vi "Ex3_BlinkingSignalLights.vi"() -> ()   [LabVIEW 2024]
panel:
  out "Array":bool[](array[boolean])
  in  "Boolean":bool
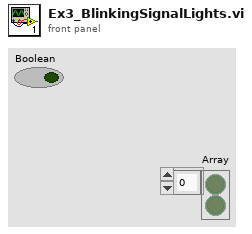
[diagram p1: front panel]
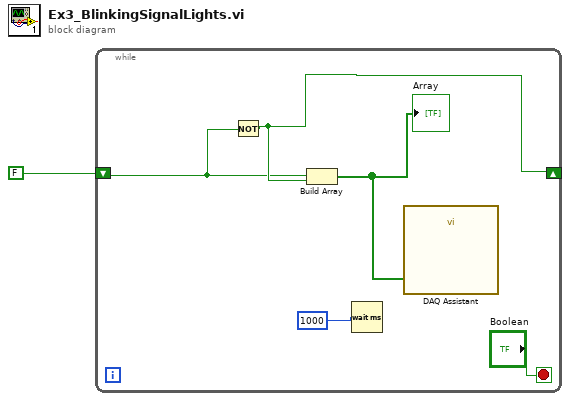
[diagram p0: block diagram]
diagram:
  n1 = while {
    shift-right: [w4] -> _
    shift-left: FALSE -> [w3]
    stop <- "Boolean" stop-if-true
    n2 = Not(x=w3) -> (.not. x?=w4:bool)
    n3 = Build Array(w3, w4) -> (w2:bool[])
    "Array" <- w2
    n4 = Wait (ms)(milliseconds to wait=u32 1000) -> ()  [unwired: 1 out]
    n5 = call "DAQ Assistant"("data"=w2) -> ()  [unwired: 17 in, 2 out]
  }
